vi "Set Bucket.vi"(8 "error in (no error)":errorcluster, 10 "Bucket name":string, 11 "Data.S3":refnum<class "LV-Data.S3.lvclass">) -> (0 "error out":errorcluster, 3 "Data.S3":refnum<class "LV-Data.S3.lvclass">)   [LabVIEW 2016, in "LV-Data.S3.lvclass"]
uses:
  LV-Data.S3.lvclass
  LV-Data.S3.lvclass/LV-Data.S3.ctl
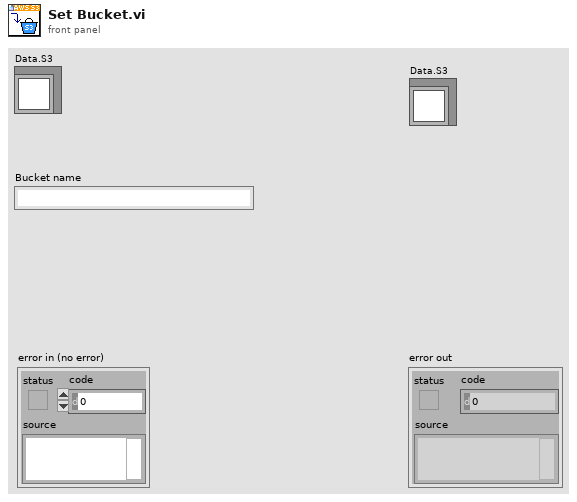
[diagram p1: front panel]
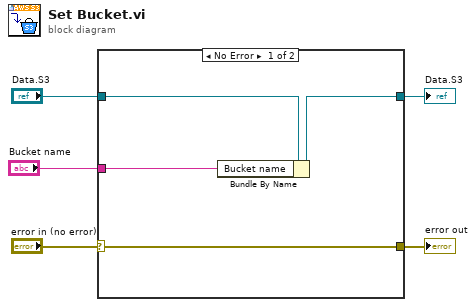
[diagram p0: block diagram]
diagram:
  n1 = case shown="No Error" "error in (no error)" {
    selector: "error in (no error)" -> [w6 w10]
    tunnel: "Data.S3" -> [w9 w11]
    tunnel: [w7 w11] -> w4
    tunnel: "Bucket name" -> [w8 _]
    tunnel: [w6 w10] -> w1
    frame No Error {
      n2 = Bundle By Name(cluster=w9, "Bucket name"=w8) -> (w7:refnum<class "LV-Data.S3.lvclass">)
    }
    frame Error {
    }
  }
  "error out" <- w1
  "Data.S3" <- w4
